vi "Init.vi"(8 "error in (no error)":errorcluster, 10 "Config Filepath":path, 11 "Scale in":refnum<class "Scale.lvclass">) -> (0 "error out":errorcluster, 2 "Read Period (sec)":dbl, 3 "Scale out":refnum<class "Scale.lvclass">)   [LabVIEW 2021, in "Scale.lvclass"]
uses:
  Scale.lvclass
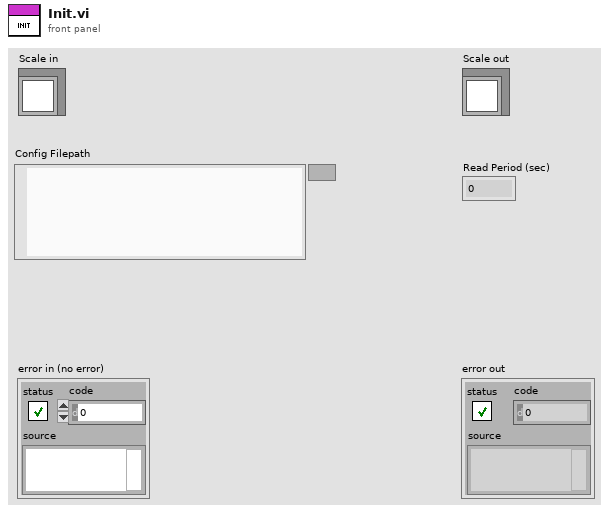
[diagram p1: front panel]
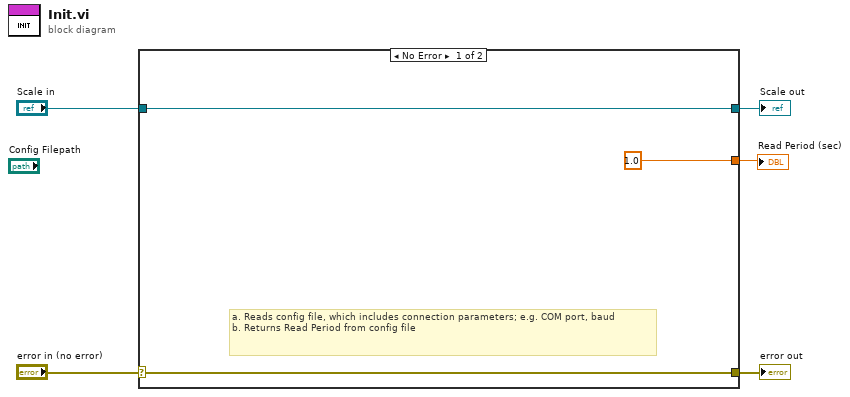
[diagram p0: block diagram]
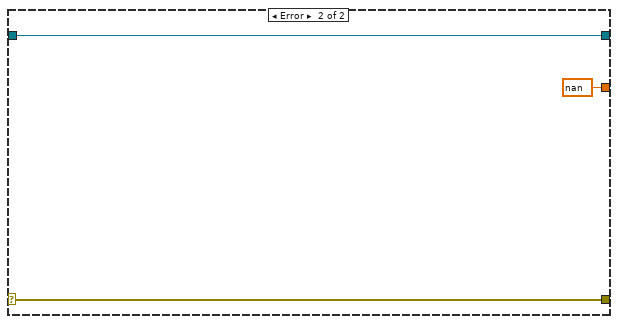
[diagram p2: hidden frame]
diagram:
  n1 = case shown="No Error" "error in (no error)" {
    selector: "error in (no error)" -> [w7 w11]
    tunnel: [w7 w11] -> w4
    tunnel: [w8 w10] -> w2
    tunnel: "Scale in" -> [w8 w10]
    tunnel: [1.0 ("Read Period (sec)") nan ("Read Period (sec)")] -> w1
    frame No Error {
      # "a.\tReads config file, which includes connection parameters; e.g. COM port, baud\nb.\tReturns Read Period from config file"
    }
    frame Error {
    }
  }
  "error out" <- w4
  "Scale out" <- w2
  "Read Period (sec)" <- w1
